vi "A 侧面 处理函数CCD5.vi"(7 "Image Name":string="I1", 8 "error in (no error)":errorcluster caption="错误输入（无错误）", 9 "相机选择":T1="cam5" caption="Session Out CCD3", 10 "New Image":T2, 11 "ParamsUI":T3={"IsNorImage"=TRUE, "Exposure Values"=100289, "ImagePath"=path "C:/Users/hedongpo/Desktop/514-hdp/Alignment Assemble System/Test Picture/B/3.bmp", "相机选择"="cam4"} caption="参数界面" {"Exposure Values" scale=0.0..200000.0}) -> (0 "error out":errorcluster caption="错误输出", 2 "Session Out":T1, 3 "Image out":T2(plugin-control), 4 "数值":dbl)   [LabVIEW 2017]
uses:
  <vilib>/userdefined/High Color/IMAQdx.ctl
  <vilib>/vision/Image Controls.llb/IMAQ Image.ctl
  <vilib>/vision/driver/IMAQdx.llb/IMAQdx Buffer Number Mode.ctl
  <resource>/objmgr/imaqdx.rc
  Global System.vi
  <vilib>/vision/driver/NI_Vision_Acquisition_Software.lvlib
  <vilib>/vision/NI_Vision_Development_Module.lvlib
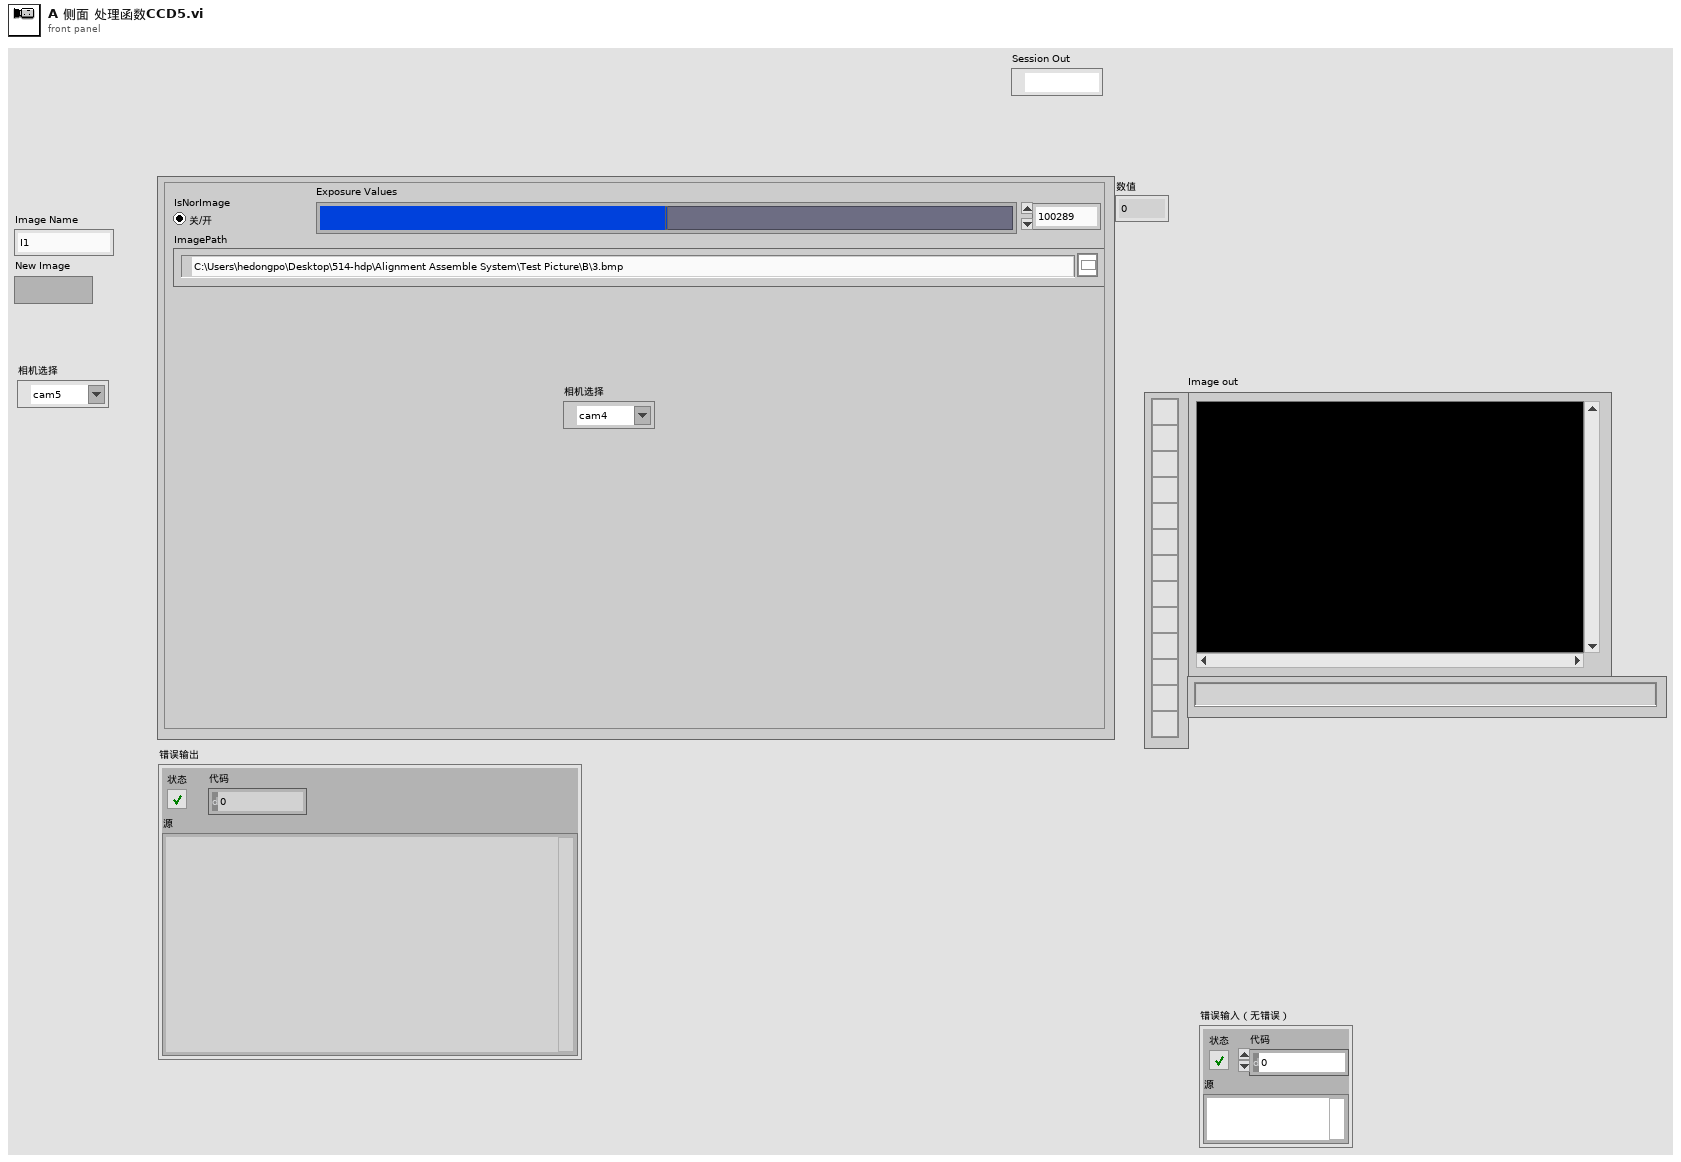
[diagram p1: front panel]
types:
  T1 = typedef "IMAQdx.ctl" = refnum<k21>
  T2 = typedef "IMAQ Image.ctl" = refnum<image>
  T3 = cluster{"IsNorImage":bool, "Exposure Values":i64, "ImagePath":path, "相机选择":T1}
  T4 = cluster{"IsNorImage":bool, "Exposure Values":u32, "ImagePath":path}
  T5 = typedef "Image Type" = u32
  T6 = typedef "NI_Vision_Acquisition_Software.lvlib/IMAQdx Buffer Number Mode.ctl" = enum32{"Next", "Last", "Buffer Number", "Every", "Last New"}
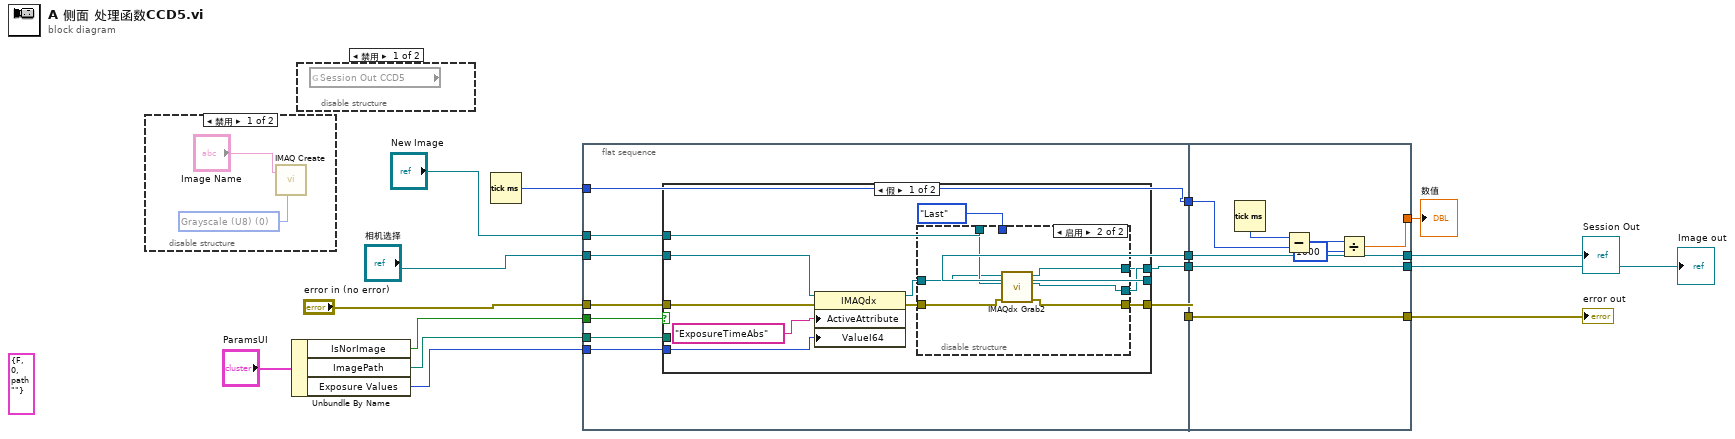
[diagram p0: block diagram]
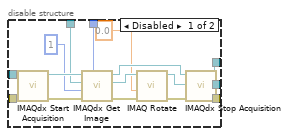
[diagram p4: hidden frame]
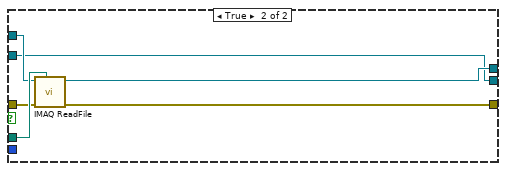
[diagram p5: hidden frame]
diagram:
  (unwired) T4 {"IsNorImage"=FALSE, "Exposure Values"=0, "ImagePath"=path ""} ("ParamsUI")
  n1 = disable-structure shown="禁用" {
    frame Disabled {
      w17 = T5 0 items=["Grayscale (U8)", "Grayscale (I16)", "Grayscale (SGL)", "Complex (CSG)", "RGB (U32)", "HSL (U32)", "RGB (U64)", "Grayscale (U16)"] ("Image Type")
      n2 = call "IMAQ Create"("Image Name"="Image Name", "Image Type"=w17) -> ()  [unwired: 3 in, 2 out]
    }
    frame Enabled {
    }
  }
  n3 = Unbundle By Name("ParamsUI") -> ("IsNorImage"=w4:bool, "ImagePath"=w3:path, "Exposure Values"=w16:i64)
  n4 = disable-structure shown="禁用" {
    frame Disabled {
      n5 = global read "Global System.vi" "Session Out CCD5"() -> ()  [unwired: 1 out]
    }
    frame Enabled {
    }
  }
  n6 = Tick Count (ms)() -> (millisecond timer value=w10:u32)
  n7 = flat-sequence {
    tunnel: w4 -> [w28]
    tunnel: w3 -> [w27]
    tunnel: w16 -> [w26]
    tunnel: "New Image" -> [w25]
    tunnel: "error in (no error)" -> [w24]
    tunnel: "相机选择" -> [w21]
    tunnel: w10 -> [w19]
    tunnel: [w23] -> w9
    tunnel: [w22] -> w8
    tunnel: [w20] -> w7
    tunnel: [w19] -> w6
    tunnel: [w72] -> w11
    tunnel: [w73] -> w12
    tunnel: [w74] -> w14
    tunnel: w9 -> [w74]
    tunnel: w8 -> [w73]
    tunnel: w7 -> [w72]
    tunnel: w6 -> [w70]
    tunnel: [w67] -> w5
    frame #0 {
      n8 = case shown="假" w28 {
        tunnel: w27 -> [_ w66]
        tunnel: [w37 w65] -> w22
        tunnel: w26 -> [w32 _]
        tunnel: w21 -> [w34 w61]
        tunnel: w25 -> [w38 w64]
        tunnel: w24 -> [w33 w63]
        tunnel: [w35 w62] -> w23
        tunnel: [w36 w61] -> w20
        frame False {
          n9 = property class="IMAQdx"(reference=w34, error in=w33, "ActiveAttribute"="ExposureTimeAbs", "ValueI64"=w32) -> (reference out=w31:T1, error out=w30:errorcluster)
          n10 = disable-structure shown="启用" {
            disable-tunnel: IMAQdx_Buffer_Number_Mode."Last" ("Buffer Number Mode (Next)") -> [w51 _]
            disable-tunnel: w38 -> [w45 w58]
            disable-tunnel: [w44 w55] -> w37
            disable-tunnel: [w43 w56] -> w36
            disable-tunnel: [w42 w59] -> w35
            disable-tunnel: w31 -> [w41 w57]
            disable-tunnel: w30 -> [w40 w60]
            frame Disabled {
              n11 = call <vilib>:"IMAQdx Start Acquisition.vi"("error in"=w40, "Session In"=w41) -> ("error out"=w53:errorcluster, "Session Out"=w54:T1)  [unwired: 8 in]
              n12 = call <vilib>:"IMAQdx Get Image.vi"("Buffer Number Mode (Next)"=w51, "error in"=w53, "Buffer Number In"=u32 1, "Image In"=w45, "Session In"=w54) -> ("error out"=w48:errorcluster, "Image Out"=w49:T2, "Session Out"=w50:T1)  [unwired: 3 in, 1 out]
              n13 = call "IMAQ Rotate"("error in (no error)"=w48, "Angle (degrees)"=sgl 0.0, "Image Src"=w49) -> ("error out"=w47:errorcluster, "Image Dst Out"=w44:T2)  [unwired: 7 in]
              n14 = call <vilib>:"IMAQdx Stop Acquisition.vi"("error in"=w47, "Session In"=w50) -> ("error out"=w42:errorcluster, "Session Out"=w43:T1)  [unwired: 8 in]
            }
            frame Enabled {
              n15 = call <vilib>:"IMAQdx Grab2.vi"("error in"=w60, "Image In"=w58, "Session In"=w57) -> ("error out"=w59:errorcluster, "Image Out"=w55:T2, "Session Out"=w56:T1)  [unwired: 5 in, 1 out]
            }
          }
        }
        frame True {
          n16 = call "IMAQ ReadFile"("File Path"=w66, "error in (no error)"=w63, "Image"=w64) -> ("error out"=w62:errorcluster, "Image Out"=w65:T2)  [unwired: 4 in, 3 out]
        }
      }
    }
    frame #1 {
      n17 = Tick Count (ms)() -> (millisecond timer value=w71:u32)
      n18 = Subtract(x=w71, y=w70) -> (x-y=w69:u32)
      n19 = Divide(x=w69, y=u32 1000) -> (x/y=w67:dbl)
    }
  }
  "Image out" <- w12
  "error out" <- w14
  "Session Out" <- w11
  "数值" <- w5
